vi "state_sensor.vi"(4 "error in":errorcluster, 7 "State sensor configuration":string=" {\n    \"type\": \"State\",\n    \"listen_port\": 8700,\n    \"desired_tags\": [\n      \"vehicle\"\n    ],\n  \"undesired_tags\": [\n  \"static\"\n  ],\n \"include_obb\": true,\n \"debug_drawing\": false\n\n}") -> (0 "error out":errorcluster, 1 "State sensor configuration":string, 2 "Raw data":string, 3 "State sensor sample":string)   [LabVIEW 2019]
doc: "Configure and read the State sensor information of the vehicle. The State sensor provides dynamic and spatial information of the elements in the scene during simulation."
uses:
  controls/Header.ctl
  tools/simx_common.vi
panel:
  out "Header":T1 {"game_time" format="%#_9g"}
  in  "state_connection":refnum<k5>
  in  "null connection":refnum<k5>
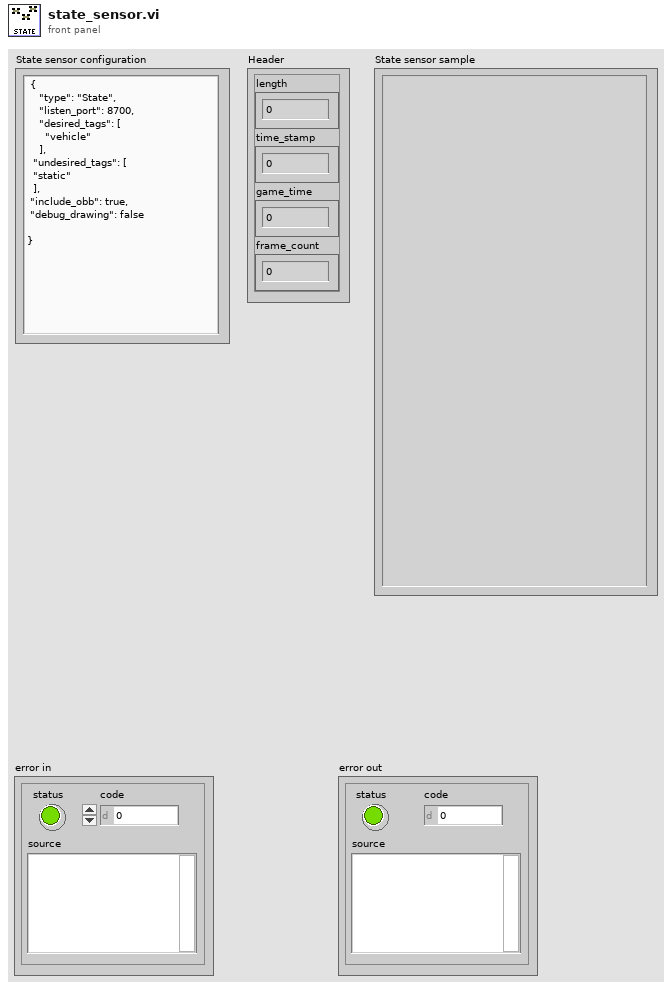
[diagram p1: front panel]
types:
  T1 = typedef "Header.ctl" = cluster{"length":u32, "time_stamp":u32, "game_time":sgl, "frame_count":u32}
  T2 = typedef "simx_connection.ctl" = cluster{"Config":T3, "Connections":T6, "Map":cluster{"lanes":cluster{"x":dbl[], "y":dbl[], "z":dbl[]}, "StartPosition":cluster{"start_points":T7, "StartRotation":dbl[], "StartLocation":dbl[]}, "Draw Map Size":T8, "DrawArea":cluster{"min_Y":dbl, "min_X":dbl, "Scale X":dbl, "Scale Y":dbl}, "Map":picture, "Map Geojson":string}}
  T3 = typedef "config.ctl" = cluster{"Trajectory":T4, "Weather":T5}
  T4 = typedef "trajectory.ctl" = cluster{"Number of frames":i32, "Frame number":i32, "Trajectory":string}
  T5 = typedef "weather.ctl" = cluster{"id":string}
  T6 = typedef "connections.ctl" = cluster{"Simulator Connection":refnum<k5>, "server_ip":string, "Port":i32, "Sensor connections":refnum<k5>[]}
  T7 = typedef "start_points.ctl" = cluster{"locations":dbl[][], "rotations":dbl[][], "type":string[]}
  T8 = typedef "LVBoundsTypeDef.ctl" = cluster{"Width":u32, "Height":u32}
  T9 = typedef "sensor_sample.ctl" = cluster{"Header":T1, "data out":string}
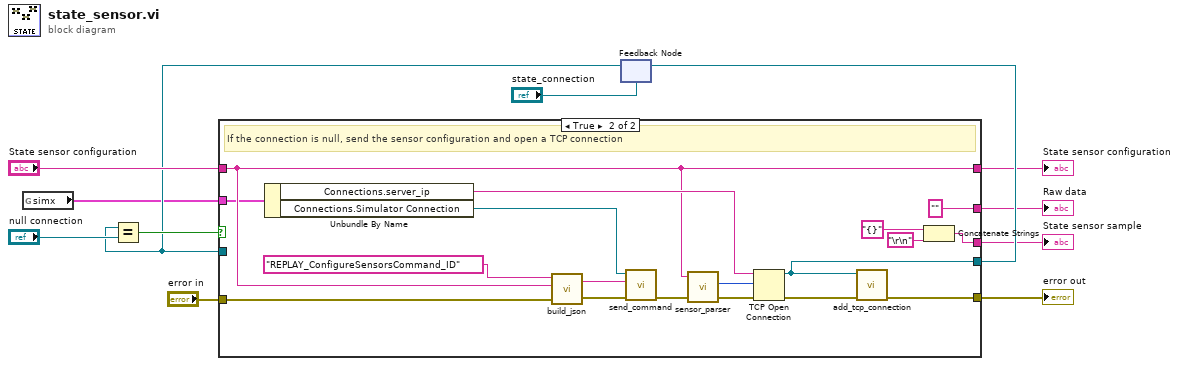
[diagram p0: block diagram]
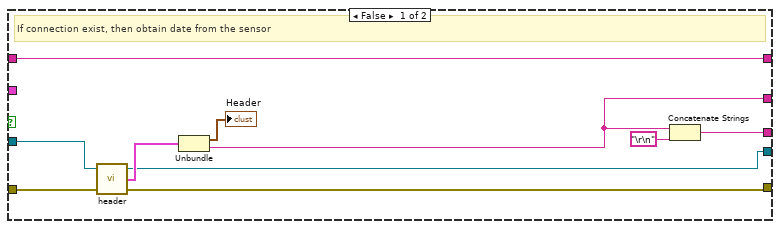
[diagram p2: hidden frame]
diagram:
  n1 = global read "simx_common.vi" "simx"() -> (w1:T2)
  n2 = feedback #1("state_connection") -> (w6:refnum<k5>)
  n3 = Equal?(x=w6, y="null connection") -> (x = y?=w8:bool)
  n4 = case shown="True" w8 {
    tunnel: [w18 w28] -> w12
    tunnel: "State sensor configuration" -> [w17 w30]
    tunnel: [w19 w27] -> w9
    tunnel: w6 -> [w22 _]
    tunnel: "error in" -> [w21 w35]
    tunnel: [w17 w30] -> w4
    tunnel: [w14 "" ("data out")] -> w3
    tunnel: [w13 w24] -> w2
    tunnel: w1 -> [_ w23]
    frame False {
      # "If connection exist, then obtain date from the sensor"
      n5 = call "header.vi"("error in"=w21, "TCP Network Connection in"=w22) -> ("error out"=w18:errorcluster, "Sensor sample"=w20:T9, "TCP Network Connection out"=w19:refnum<k5>)  [unwired: 1 in]
      n6 = Unbundle(w20) -> ("Header"=→"Header":T1, "data out"=w14:string)
      n7 = Concatenate Strings(w14, "\r\n") -> (w13:string)
    }
    frame True {
      # "If the connection is null, send the sensor configuration and open a TCP connection"
      n8 = Unbundle By Name(w23) -> ("Connections.server_ip"=w32:string, "Connections.Simulator Connection"=w33:refnum<k5>)
      n9 = call "build_json.vi"("error in"=w35, "Message"=w30, "Command_ID"="REPLAY_ConfigureSensorsCommand_ID") -> ("error out"=w38:errorcluster, "JSON Out"=w39:string)  [unwired: 1 in]
      n10 = call "send_command.vi"("error in"=w38, "JSON Command"=w39, "TCP Network Connection in"=w33) -> ("error out"=w37:errorcluster)  [unwired: 1 in, 3 out]
      n11 = call "sensor_parser.vi"("Sensor configuration"=w30, "error in"=w37) -> ("Port out"=w29:u16, "error out"=w31:errorcluster)  [unwired: 1 in, 2 out]
      n12 = TCP Open Connection(address=w32, remote port or service name=w29, error in (no error)=w31) -> (connection ID=w27:refnum<k5>, error out=w36:errorcluster)  [unwired: 2 in]
      n13 = call "add_tcp_connection.vi"("error in"=w36, "Sensor connection"=w27) -> ("error out"=w28:errorcluster)  [unwired: 5 in]
      n14 = Concatenate Strings("{}" ("data out"), "\r\n") -> (w24:string)
    }
  }
  "error out" <- w12
  "State sensor sample" <- w2
  "State sensor configuration" <- w4
  "Raw data" <- w3
  n15 = feedback-in #1(w9) -> ()
